vi "_JKISMQFGV.vi"(6 "Enum":T2, 8 "Error in":errorcluster caption="Error in (no error)", 9 "create if not found? (T)":bool=TRUE, 11 "Name(\"\" to use uuid) in":string) -> (0 "Error out":errorcluster, 2 "Name":string[](array[string]), 3 "Array":T1[](array[typedef]))   [LabVIEW 2014, in "JKI-State-Machine-Plus.lvlib"]
uses:
  JKI-State-Machine-Plus.lvlib
  _JKISMQFGVOPER.ctl
  _JKISMQ.ctl
  _Cross JKI StateMachine State Data.ctl
  _Cross JKI StateMachine State Response.ctl
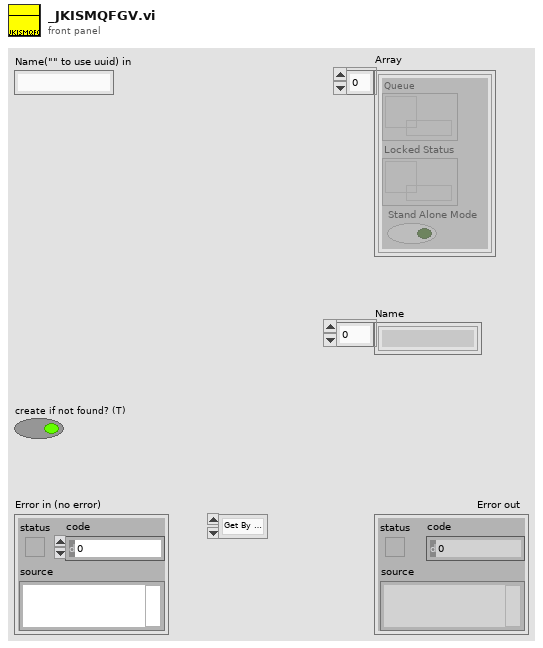
[diagram p1: front panel]
types:
  T1 = typedef "JKI-State-Machine-Plus.lvlib/_JKISMQ.ctl" = cluster{"Queue":refnum<queue>, "Locked Status":refnum<data-value>, "Stand Alone Mode":bool}
  T2 = typedef "JKI-State-Machine-Plus.lvlib/_JKISMQFGVOPER.ctl" = enum16{"Get By Name", "List"}
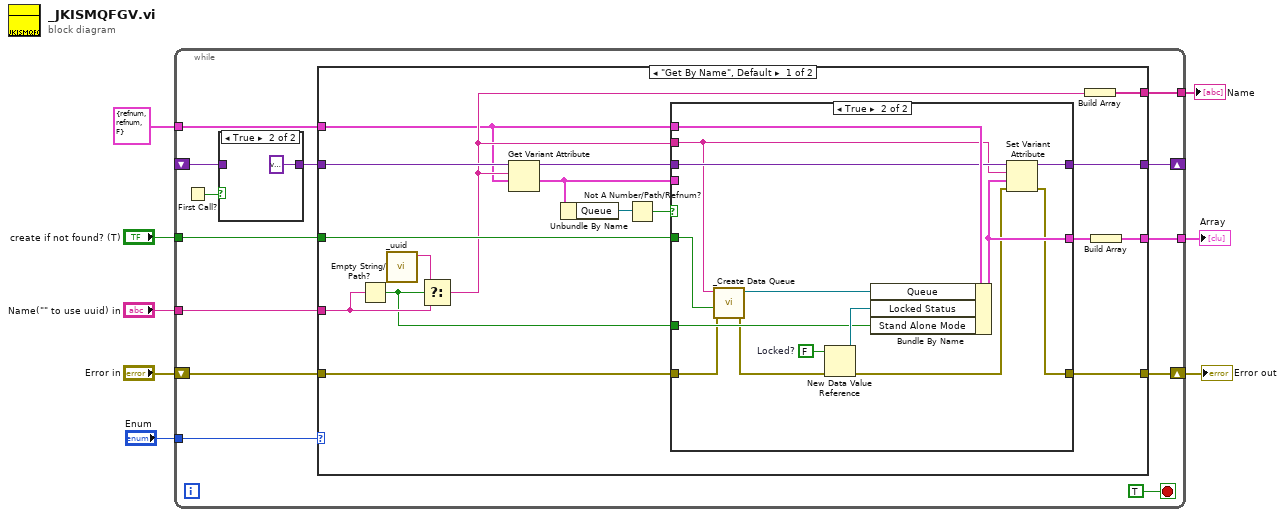
[diagram p0: block diagram]
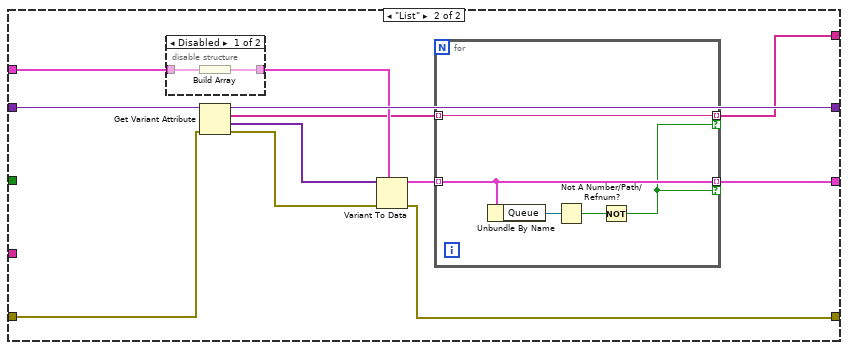
[diagram p4: hidden frame]
diagram:
  n1 = while {
    tunnel: "Enum" -> [w20]
    tunnel: "Name(\"\" to use uuid) in" -> [w19]
    tunnel: "create if not found? (T)" -> [w18]
    tunnel: [w17] -> w1
    shift-right: [w13] -> _
    shift-left: _ -> [w15]
    shift-right: [w11] -> w4
    shift-left: "Error in" -> [w12]
    tunnel: [w10] -> w3
    tunnel: T1 {"Queue"=refnum, "Locked Status"=refnum, "Stand Alone Mode"=FALSE} ("JKISMQ") -> [w9]
    stop <- TRUE stop-if-true
    n2 = First Call?() -> (First Call?: T/F=w16:bool)
    n3 = case shown="True" w16 {
      tunnel: [w22 variant] -> w14
      tunnel: w15 -> [w22 _]
      frame False {
      }
      frame True {
      }
    }
    n4 = case shown="\"Get By Name\", Default" w20 {
      tunnel: w19 -> [w39 _]
      tunnel: w18 -> [w38 _]
      tunnel: [w25 w61] -> w17
      tunnel: w14 -> [w35 w69]
      tunnel: [w33 w68] -> w13
      tunnel: w12 -> [w29 w59]
      tunnel: [w28 w58] -> w11
      tunnel: [w24 w62] -> w10
      tunnel: w9 -> [w26 w66]
      frame "Get By Name", Default {
        n5 = Empty String/Path?(string/path=w39) -> (empty?=w37:bool)
        n6 = call "_uuid.vi"() -> ("UUID"=w40:string)  [unwired: 11 in]
        n7 = Select(t=w40, s=w37, f=w39) -> (s? t:f=w27:string)
        n8 = Get Variant Attribute(Variant=w35, name=w27, default value (empty Variant)=w26) -> (duplicate Variant=w34:variant, value=w32:T1)  [unwired: 1 in, 2 out]
        n9 = Unbundle By Name(w32) -> ("Queue"=w31:refnum<queue>)
        n10 = Not A Number/Path/Refnum?(number/path/refnum=w31) -> (NaN/Path/Refnum?=w30:bool)
        n11 = case shown="True" w30 {
          tunnel: w38 -> [_ w56]
          tunnel: w37 -> [_ w53]
          tunnel: [w42 w48] -> w36
          tunnel: w27 -> [_ w49]
          tunnel: w26 -> [_ w52]
          tunnel: w34 -> [w43 w51]
          tunnel: [w43 w50] -> w33
          tunnel: w32 -> [w42 _]
          tunnel: w29 -> [w41 w47]
          tunnel: [w41 w44] -> w28
          frame False {
          }
          frame True {
            w57 = FALSE  # Locked?
            n12 = call "_Create Data Queue.vi"("error in (no error)"=w47, "create if not found? (T)"=w56, "Name"=w49) -> ("error out"=w46:errorcluster, "Queue out"=w55:refnum<queue>)  [unwired: 6 in, 1 out]
            n13 = New Data Value Reference(data value=w57, error in=w46) -> (data value reference=w54:refnum<data-value>, error out=w45:errorcluster)
            n14 = Bundle By Name(cluster=w52, "Queue"=w55, "Locked Status"=w54, "Stand Alone Mode"=w53) -> (w48:T1)
            n15 = Set Variant Attribute(Variant=w51, name=w49, value=w48, error in=w45) -> (Variant out=w50:variant, error out=w44:errorcluster)  [unwired: 1 out]
          }
        }
        n16 = Build Array(w27) -> (w24:string[])
        n17 = Build Array(w36) -> (w25:T1[])
      }
      frame "List" {
        n18 = disable-structure shown="Disabled" {
          disable-tunnel: w66 -> [w76 _]
          disable-tunnel: [w75 _] -> w65
          frame Disabled {
            n19 = Build Array(w76) -> (w75:T1[])
          }
          frame Enabled {
          }
        }
        n20 = Get Variant Attribute(Variant=w69, error in=w59) -> (duplicate Variant=w68:variant, names=w63:string[], values=w67:variant[], error out=w60:errorcluster)  [unwired: 2 in]
        n21 = Variant To Data(error in=w60, type=w65, Variant=w67) -> (data=w64:T1[], error out=w58:errorcluster)
        n22 = for {
          tunnel: w64 -> [w73] mode=indexing
          tunnel: w63 -> [w74] mode=indexing
          tunnel: [w74] -> w62 mode=indexing if=w70
          tunnel: [w73] -> w61 mode=indexing if=w70
          n23 = Unbundle By Name(w73) -> ("Queue"=w72:refnum<queue>)
          n24 = Not A Number/Path/Refnum?(number/path/refnum=w72) -> (NaN/Path/Refnum?=w71:bool)
          n25 = Not(x=w71) -> (.not. x?=w70:bool)
        }
      }
    }
  }
  "Error out" <- w4
  "Name" <- w3
  "Array" <- w1
